vi "Add DAQ Hardware_Add Counters.vi"(8 "error in (no error)":errorcluster, 9 "Counter Settings":T4 {"Position Measurements"."ZIndexMode" items=["AHighBHigh"=10040, "AHighBLow"=10041, "ALowBHigh"=10042, "ALowBLow"=10043]; "Position Measurements"."Decoding" items=["Decoding1X"=10090, "Decoding2X"=10091, "Decoding4X"=10092, "DecodingPulseCounting"=10313]; "Count Measurements"."CountDirection" items=["Down"=10124, "Up"=10128, "ExternallyControlled"=10326]; "Count Measurements"."Edge" items=["Falling"=10171, "Rising"=10280]; "Period Measurements"."Edge" items=["Falling"=10171, "Rising"=10280]; "Frequency Measurements"."Edge" items=["Falling"=10171, "Rising"=10280]}, 11 "DAQ Ref":refnum<k24>) -> (0 "error out":errorcluster, 3 "DAQ Ref Out":refnum<k24>)   [LabVIEW 2019, in "Simple SysDef API.lvlib"]
uses:
  <userlib>/SimpleSysDef/Simple SysDef API.lvlib
  NationalInstruments.VeriStand.SystemDefinitionAPI
  <userlib>/SimpleSysDef/_SubVIs/Add Frequency Measurement Channels_Settings.ctl
  <userlib>/SimpleSysDef/_SubVIs/Add Count Measurement Channels_Settings.ctl
  <userlib>/SimpleSysDef/_SubVIs/Add Position Measurement Channels_Settings.ctl
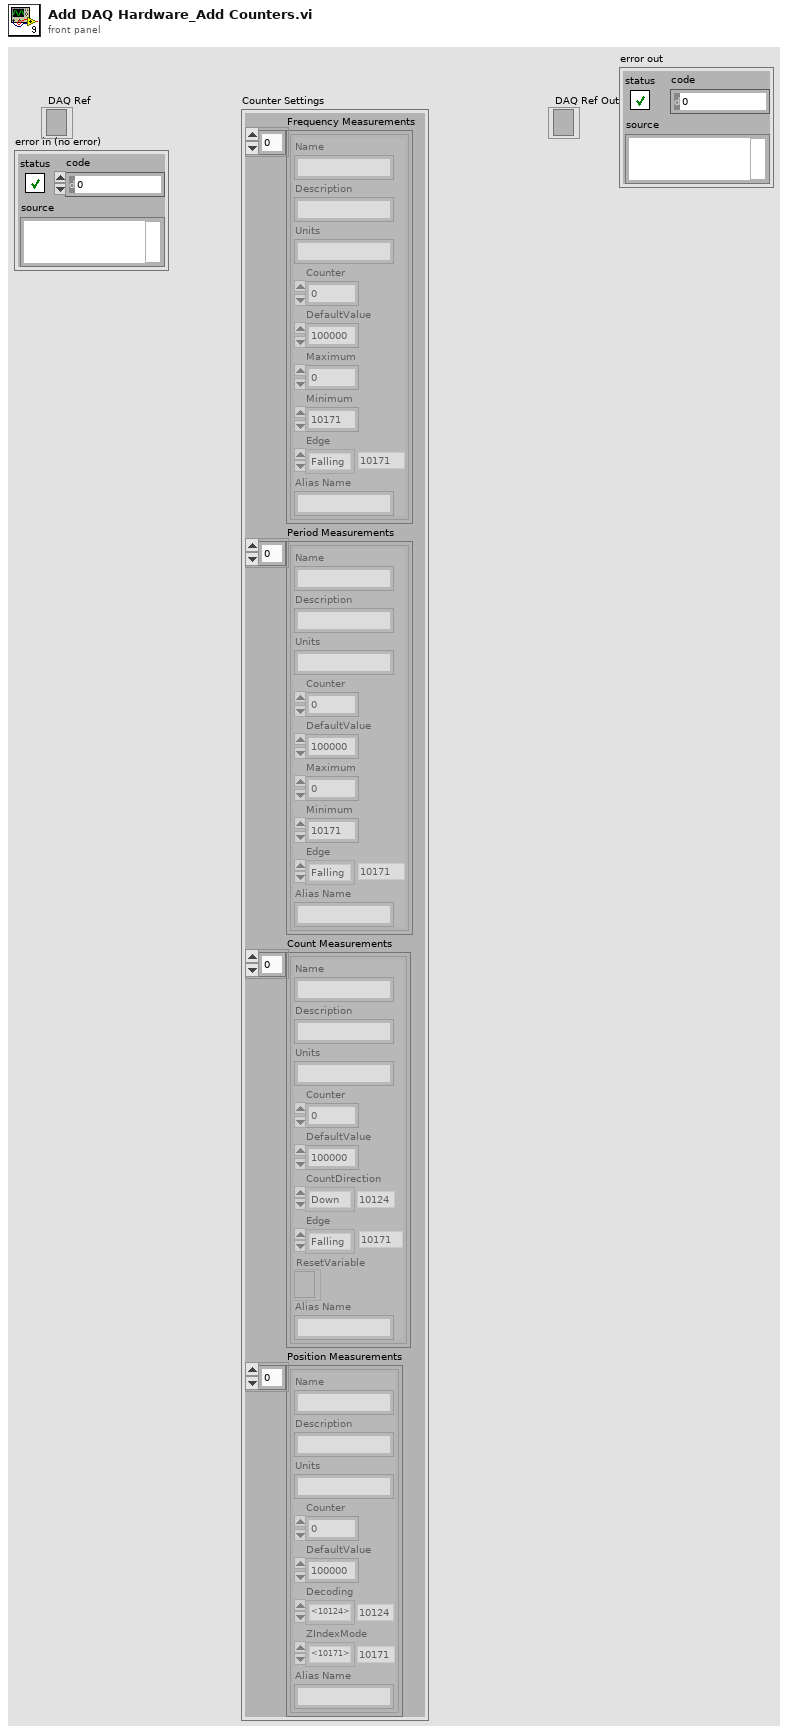
[diagram p1: front panel]
types:
  T1 = typedef "Simple SysDef API.lvlib/Add Frequency Measurement Channels_Settings.ctl" = cluster{"Name":string, "Description":string, "Units":string, "Counter":u32, "DefaultValue":dbl, "Maximum":dbl, "Minimum":dbl, "Edge":i32, "Alias Name":string}
  T2 = typedef "Simple SysDef API.lvlib/Add Count Measurement Channels_Settings.ctl" = cluster{"Name":string, "Description":string, "Units":string, "Counter":u32, "DefaultValue":dbl, "CountDirection":i32, "Edge":i32, "ResetVariable":refnum<k24>, "Alias Name":string}
  T3 = typedef "Simple SysDef API.lvlib/Add Position Measurement Channels_Settings.ctl" = cluster{"Name":string, "Description":string, "Units":string, "Counter":u32, "DefaultValue":dbl, "Decoding":i32, "ZIndexMode":i32, "Alias Name":string}
  T4 = cluster{"Frequency Measurements":T1[], "Period Measurements":T1[], "Count Measurements":T2[], "Position Measurements":T3[]}
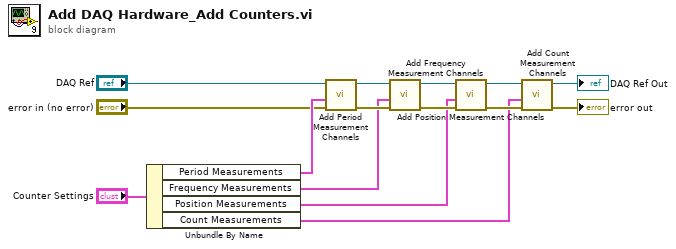
[diagram p0: block diagram]
diagram:
  n1 = Unbundle By Name("Counter Settings") -> ("Period Measurements"=w6:T1[], "Frequency Measurements"=w5:T1[], "Position Measurements"=w4:T3[], "Count Measurements"=w3:T2[])
  n2 = call <userlib>:"Add Period Measurement Channels.vi"("error in (no error)"="error in (no error)", "Period Measurement"=w6, "DAQ Ref"="DAQ Ref") -> ("error out"=w12:errorcluster, "DAQ Ref"=w13:refnum<k24>)  [unwired: 7 in]
  n3 = call <userlib>:"Add Frequency Measurement Channels.vi"("error in (no error)"=w12, "Frequency Measurement"=w5, "DAQ Ref"=w13) -> ("error out"=w11:errorcluster, "DAQ Ref"=w14:refnum<k24>)  [unwired: 7 in]
  n4 = call <userlib>:"Add Position Measurement Channels.vi"("error in (no error)"=w11, "Position Measurement"=w4, "DAQ Ref"=w14) -> ("error out"=w10:errorcluster, "DAQ Ref"=w15:refnum<k24>)  [unwired: 7 in]
  n5 = call <userlib>:"Add Count Measurement Channels.vi"("error in (no error)"=w10, "Count Measurement"=w3, "DAQ Ref"=w15) -> ("error out"=→"error out":errorcluster, "DAQ Ref"=→"DAQ Ref Out":refnum<k24>)  [unwired: 7 in]
